vi "短日期时间转长日期格式.vi"(10 "table输入":string(combo), 11 "data":string[][](table)) -> (3 "输出数组":string[][](array[string]))   [LabVIEW 2016]
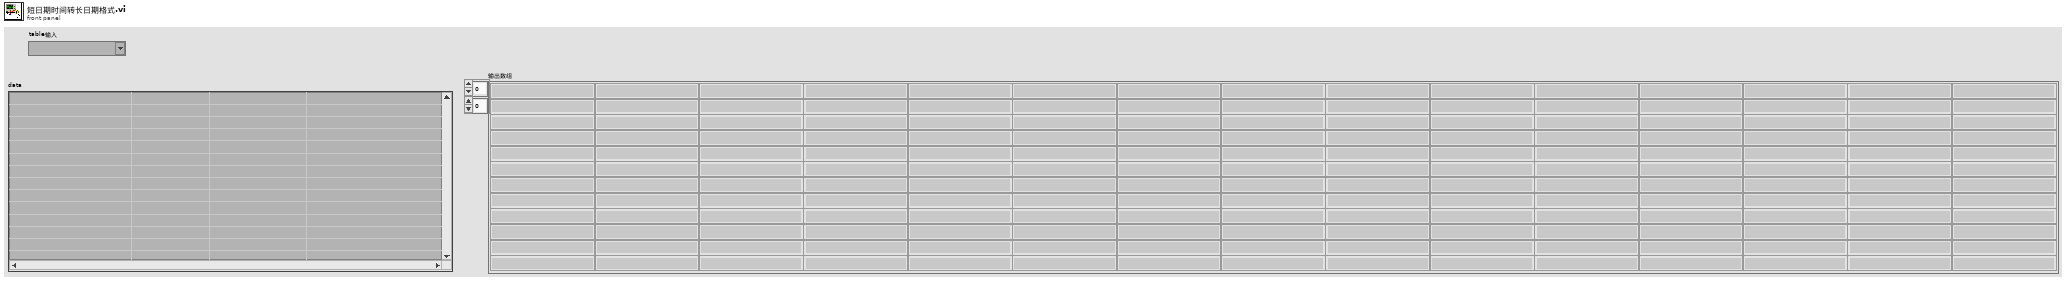
[diagram p1: front panel]
types:
  T1 = typedef "LVDateTimeRec.ctl" = cluster{"秒数的小数部分":dbl, "秒":i32, "分":i32, "时":i32, "日":i32, "月":i32, "年":i32, "天数（周）":i32, "天数（年）":i32, "DST":i32}
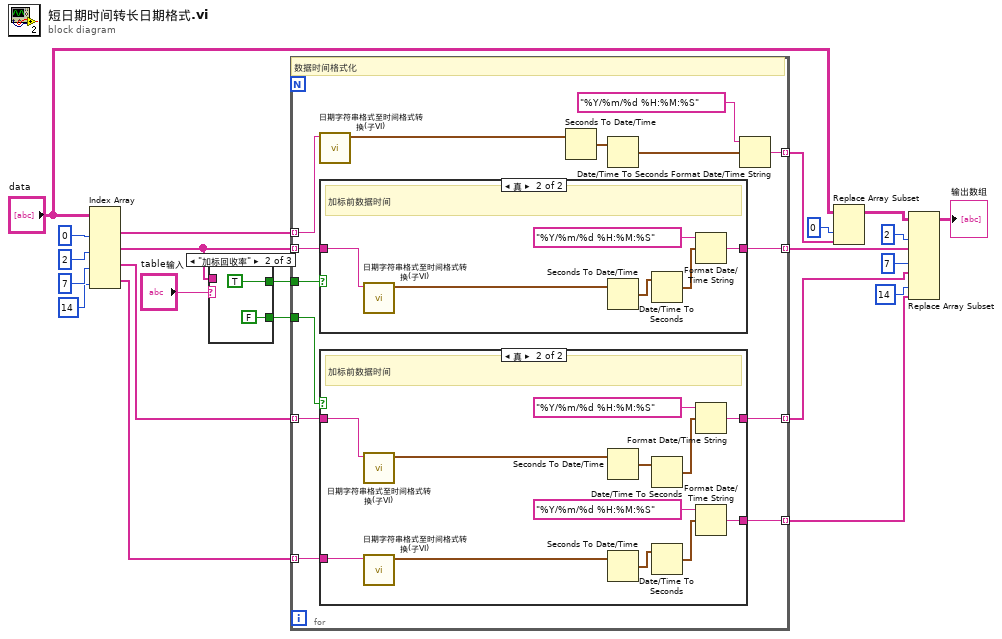
[diagram p0: block diagram]
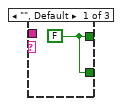
[diagram p4: hidden frame]
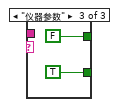
[diagram p5: hidden frame]
diagram:
  n1 = Index Array(array="data", index (col) #1=0 ("禁用的索引 (列)"), index (col) #2=2 ("索引 (列)"), index (col) #3=7 ("索引 (列)"), index (col) #4=14 ("索引 (列)")) -> (element #1=w19:string[], element #2=w18:string[], element #3=w6:string[], element #4=w5:string[])  [unwired: 4 in]
  n2 = case shown="\"加标回收率\"" "table输入" {
    tunnel: [w23 TRUE FALSE] -> w17
    tunnel: w18 -> [_ _ _]
    tunnel: [w23 FALSE TRUE] -> w9
    frame "", Default {
      w23 = FALSE
    }
    frame "加标回收率" {
    }
    frame "仪器参数" {
    }
  }
  n3 = for "For循环" {
    tunnel: w19 -> [w36] mode=indexing
    tunnel: w18 -> [w35] mode=indexing
    tunnel: w17 -> [w41]
    tunnel: [w34] -> w15 mode=indexing
    tunnel: [w33] -> w12 mode=indexing
    tunnel: w9 -> [w32]
    tunnel: w6 -> [w31] mode=indexing
    tunnel: w5 -> [w30] mode=indexing
    tunnel: [w29] -> w2 mode=indexing
    tunnel: [w28] -> w1 mode=indexing
    # "数据时间格式化"
    n4 = call "日期字符串格式至时间格式转换(子VI).vi"("data[0]"=w36) -> ("time stamp"=w39:timestamp)  [unwired: 10 in]
    n5 = case shown="真" w41 {
      tunnel: w35 -> [w56 w58]
      tunnel: [w56 w57] -> w33
      frame False {
      }
      frame True {
        # "加标前数据时间"
        n6 = call "日期字符串格式至时间格式转换(子VI).vi"("data[0]"=w58) -> ("time stamp"=w60:timestamp)  [unwired: 10 in]
        n7 = Seconds To Date/Time(time stamp (now)=w60) -> (date time rec=w59:T1)  [unwired: 1 in]
        n8 = Date/Time To Seconds(2:w59) -> (0:w61:timestamp)  [unwired: 1 in]
        n9 = Format Date/Time String(time format string (%c)="%Y/%m/%d %H:%M:%S" ("时间格式字符串(%c)"), seconds (now)=w61) -> (date/time string=w57:string)  [unwired: 1 in]
      }
    }
    n10 = case shown="真" w32 {
      tunnel: w31 -> [w43 w51]
      tunnel: [w43 w50] -> w29
      tunnel: w30 -> [w42 w45]
      tunnel: [w42 w44] -> w28
      frame False {
      }
      frame True {
        # "加标前数据时间"
        n11 = call "日期字符串格式至时间格式转换(子VI).vi"("data[0]"=w51) -> ("time stamp"=w53:timestamp)  [unwired: 10 in]
        n12 = call "日期字符串格式至时间格式转换(子VI).vi"("data[0]"=w45) -> ("time stamp"=w48:timestamp)  [unwired: 10 in]
        n13 = Seconds To Date/Time(time stamp (now)=w53) -> (date time rec=w52:T1)  [unwired: 1 in]
        n14 = Seconds To Date/Time(time stamp (now)=w48) -> (date time rec=w49:T1)  [unwired: 1 in]
        n15 = Date/Time To Seconds(2:w52) -> (0:w54:timestamp)  [unwired: 1 in]
        n16 = Date/Time To Seconds(2:w49) -> (0:w47:timestamp)  [unwired: 1 in]
        n17 = Format Date/Time String(time format string (%c)="%Y/%m/%d %H:%M:%S" ("时间格式字符串(%c)"), seconds (now)=w54) -> (date/time string=w50:string)  [unwired: 1 in]
        n18 = Format Date/Time String(time format string (%c)="%Y/%m/%d %H:%M:%S" ("时间格式字符串(%c)"), seconds (now)=w47) -> (date/time string=w44:string)  [unwired: 1 in]
      }
    }
    n19 = Seconds To Date/Time(time stamp (now)=w39) -> (date time rec=w40:T1)  [unwired: 1 in]
    n20 = Date/Time To Seconds(2:w40) -> (0:w38:timestamp)  [unwired: 1 in]
    n21 = Format Date/Time String(time format string (%c)="%Y/%m/%d %H:%M:%S" ("时间格式字符串(%c)"), seconds (now)=w38) -> (date/time string=w34:string)  [unwired: 1 in]
  }
  n22 = Replace Array Subset(array="data", new element=w15, index (col)=0 ("禁用的索引 (列)")) -> (w11:string[][])  [unwired: 1 in]
  n23 = Replace Array Subset(array=w11, new element #1=w12, index (col) #1=2 ("索引 (列)"), new element #2=w2, index (col) #2=7 ("索引 (列)"), new element #3=w1, index (col) #3=14 ("索引 (列)")) -> (→"输出数组":string[][])  [unwired: 3 in]
